vi "Analog Read.vi"() -> ()   [LabVIEW 2018]
uses:
  <vilib>/myRIO/Common/Instrument Driver Framework/myRIO v1.0/AI/typedefs/AI Channels List.ctl
  <vilib>/myRIO/Common/Instrument Driver Framework/myRIO v1.0/AI/typedefs/AI Channels Enum.ctl
panel:
  out "error out":errorcluster
  out "Timestamp":u32
  out "NavX Output":T1
  in  "error in (no error)":errorcluster
  in  "Zero Yaw":bool
  out "Numeric":dbl
  out "Scaled Signals":dbl
  out "element":dbl
  in  "stop":bool
  out "Array":dbl[](array[numeric])
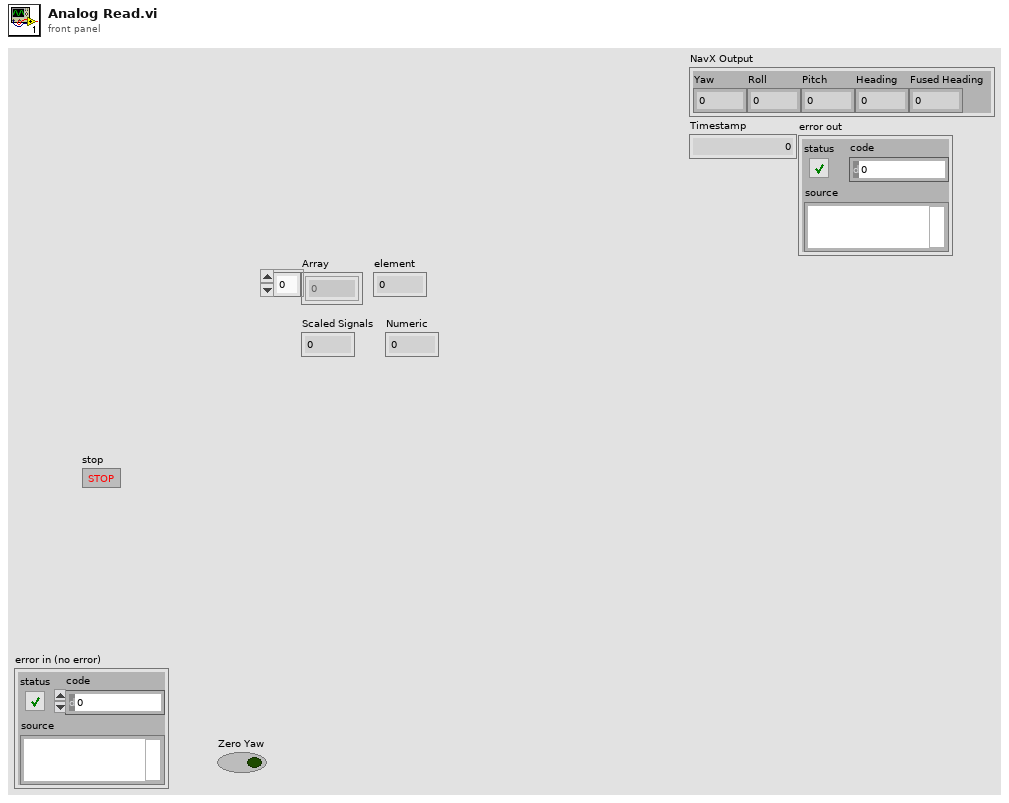
[diagram p1: front panel]
types:
  T1 = cluster{"Yaw":dbl, "Roll":dbl, "Pitch":dbl, "Heading":dbl, "Fused Heading":dbl}
  T2 = typedef "AI Channels List.ctl" = T3[]
  T3 = typedef "AI Channels Enum.ctl" = enum16{"Not Connected", "AudioIn/Left", "AudioIn/Right", "C/AI0", "C/AI1", "A/AI0", "A/AI1", "A/AI2", "A/AI3", "A/AI4", "A/AI5", "A/AI6", "A/AI7", "B/AI0", "B/AI1", "B/AI2", "B/AI3", "B/AI4", "B/AI5", "B/AI6", "B/AI7", "AI/AI0", "AI/AI1", "AI/AI2", "AI/AI3", "A/AI0 (DIFF)", "A/AI1 (DIFF)", "A/AI2 (DIFF)", "A/AI3 (DIFF)", "B/AI0 (DIFF)", "B/AI1 (DIFF)", "B/AI2 (DIFF)", "B/AI3 (DIFF)"}
  T4 = typedef "Analog Scaling Constants List.ctl" = T5[]
  T5 = typedef "Analog Scaling Constants.ctl" = cluster{"LSB Weight (Volts)":dbl, "Offset (Volts)":dbl, "Signed?":bool}
  T6 = cluster{"Scale Constants Array":T4, "FPGA Reference Out":refnum<k20>, "AI Channel":T2}
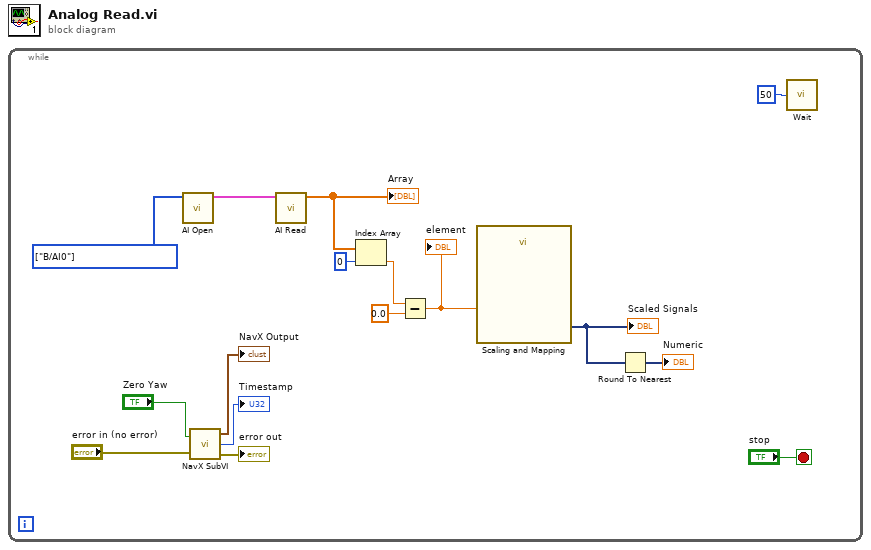
[diagram p0: block diagram]
diagram:
  n1 = while {
    stop <- "stop" stop-if-true
    w16 = T2 [enum."B/AI0"] items=["Not Connected", "AudioIn/Left", "AudioIn/Right", "C/AI0", "C/AI1", "A/AI0", "A/AI1", "A/AI2", "A/AI3", "A/AI4", "A/AI5", "A/AI6", "A/AI7", "B/AI0", "B/AI1", "B/AI2", "B/AI3", "B/AI4", "B/AI5", "B/AI6", "B/AI7", "AI/AI0", "AI/AI1", "AI/AI2", "AI/AI3", "A/AI0 (DIFF)", "A/AI1 (DIFF)", "A/AI2 (DIFF)", "A/AI3 (DIFF)", "B/AI0 (DIFF)", "B/AI1 (DIFF)", "B/AI2 (DIFF)", "B/AI3 (DIFF)"] ("AI Channel")
    n2 = call <vilib>:"AI Open.vi"("AI Channel"=w16) -> ("Analog Info"=w15:T6)  [unwired: 9 in, 1 out]
    n3 = call "NavX SubVI.vi"("Zero Yaw"="Zero Yaw", "error in (no error)"="error in (no error)") -> ("NavX Output"=→"NavX Output":T1, "Timestamp"=→"Timestamp":u32, "error out"=→"error out":errorcluster)
    n4 = call <vilib>:"AI Read.vi"("Analog Info"=w15) -> ("Array"=w13:dbl[])  [unwired: 9 in, 1 out]
    "Array" <- w13
    n5 = Index Array(array=w13, index=0) -> (element=w8:dbl)
    n6 = Subtract(x=w8, y=0.0) -> (x-y=w9:dbl)
    "element" <- w9
    n7 = call "Scaling and Mapping"("Signals"=w9) -> ("Scaled Signals"=w11:dynamicdata)  [unwired: 9 in, 1 out]
    "Scaled Signals" <- w11
    n8 = Round To Nearest(number=w11) -> (nearest integer value=→"Numeric":dynamicdata)
    n9 = call "Wait"("Count(mSec)"=u32 50) -> ()  [unwired: 1 out]
  }
